vi "sub_write_custom_pads.vi"(11 "input string":string) -> (3 "result string":string)   [LabVIEW 2016]
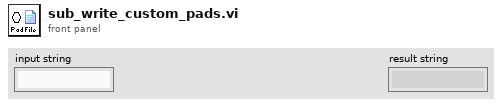
[diagram p1: front panel]
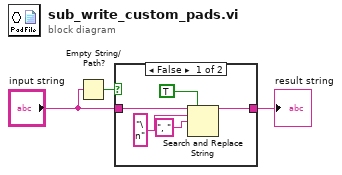
[diagram p0: block diagram]
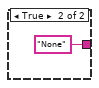
[diagram p2: hidden frame]
diagram:
  n1 = Empty String/Path?(string/path="input string") -> (empty?=w1:bool)
  n2 = case shown="False" w1 {
    tunnel: [w6 "None" ("result string")] -> w3
    tunnel: "input string" -> [w4 _]
    frame False {
      n3 = Search and Replace String(replace all?=TRUE ("replace all? (F)"), input string=w4, search string="\n", replace string=", " ("replace string (\"\")")) -> (result string=w6:string)  [unwired: 4 in, 3 out]
    }
    frame True {
    }
  }
  "result string" <- w3
